vi "FilterModeString.vi"(8 "error in (no error)":errorcluster, 11 "FilterMode":T1) -> (0 "error out":errorcluster, 3 "FilterModeString":string)   [LabVIEW 2026, in "Lumberjack.lvlib"]
uses:
  Lumberjack.lvlib
  TypeDefs/FilterMode.ctl
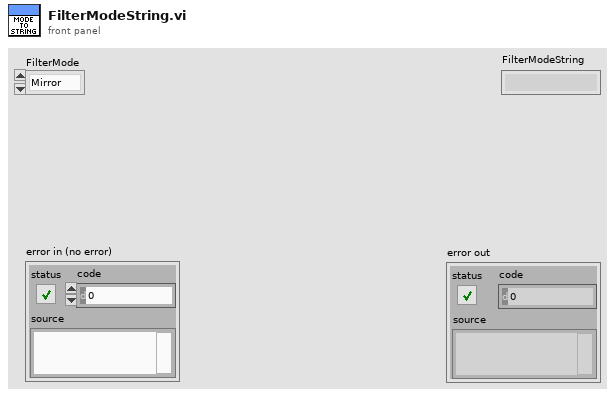
[diagram p1: front panel]
types:
  T1 = typedef "Lumberjack.lvlib/FilterMode.ctl" = enum16{"Mirror", "Routed"}
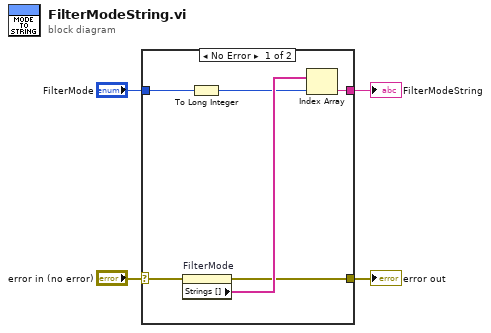
[diagram p0: block diagram]
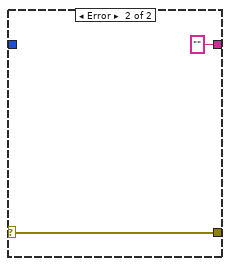
[diagram p2: hidden frame]
diagram:
  n1 = case shown="No Error" "error in (no error)" {
    selector: "error in (no error)" -> [w5 w12]
    tunnel: [w8 ""] -> w2
    tunnel: [w7 w12] -> w3
    tunnel: "FilterMode" -> [w6 _]
    frame No Error {
      n2 = property on="FilterMode" class="Enum (strict)"(error in=w5) -> (error out=w7:errorcluster, "Strings []"=w10:string[])  [unwired: 1 in, 1 out]
      n3 = To Long Integer(number=w6) -> (32bit integer=w9:i32)
      n4 = Index Array(array=w10, index=w9) -> (element=w8:string)
    }
    frame Error {
    }
  }
  "error out" <- w3
  "FilterModeString" <- w2
